vi "ws_set HTTP header for export.vi"(8 "error in (no error)":errorcluster, 9 "Content-type (\"application/octet-stream\")":string="application/octet-stream", 10 "filename (\"\")":string, 11 "httpRequestID":u32) -> (0 "error out":errorcluster)   [LabVIEW 2011]
uses:
  <vilib>/wsapi/NI_WebServices.lvlib
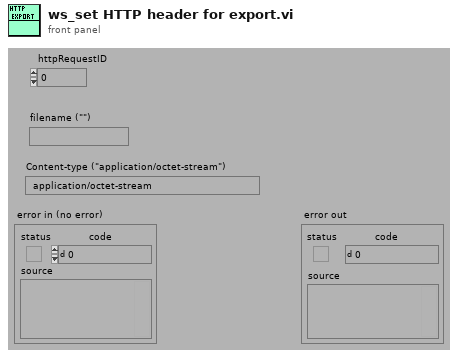
[diagram p1: front panel]
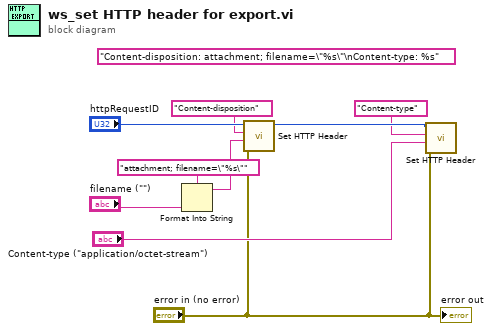
[diagram p0: block diagram]
diagram:
  (unwired) "Content-disposition: attachment; filename=\"%s\"\nContent-type: %s"
  n1 = Format Into String(format string="attachment; filename=\"%s\"" ("header value"), "filename (\"\")") -> (resulting string=w5:string)  [unwired: 2 in, 1 out]
  n2 = call <vilib>:"Set HTTP Header.vi"("error in (no error)"="error in (no error)", "header value"=w5, "header"="Content-disposition", "httpRequestID"="httpRequestID") -> ("httpRequestID out"=w7:u32)  [unwired: 6 in, 1 out]
  n3 = call <vilib>:"Set HTTP Header.vi"("error in (no error)"="error in (no error)", "header value"="Content-type (\"application/octet-stream\")", "header"="Content-type", "httpRequestID"=w7) -> ()  [unwired: 6 in, 2 out]
  "error out" <- "error in (no error)"
